vi "Begin.vi"(8 "error in":errorcluster) -> (0 "error out":errorcluster)   [LabVIEW 2016]
doc: "Called before other user functions, this VI is expected to open initial I/O refnums, load in file data, and do all program initialization. Notice that the <B>error out</B> terminal is simply used for data flow. Wiring it to other structures or subVIs ensures that this VI runs first."
uses:
  <vilib>/Rock Robotics/WPI/Joystick/WPI_JoystickDeviceEnum.ctl
  <vilib>/Rock Robotics/SystemInterfaces/DIO/FPGA_DIOPWMChannel.ctl
  <vilib>/Rock Robotics/WPI/SafetyOutput/WPI_SafetyOutputConfigMenu.ctl
  <vilib>/Rock Robotics/SystemInterfaces/DIO/FPGA_DIOChannel.ctl
  <vilib>/Rock Robotics/WPI/Solenoid/WPI_SolenoidChannel.ctl
  <vilib>/Rock Robotics/SystemInterfaces/i2clib/i2c_bus.ctl
  <vilib>/Rock Robotics/WPI/SerialPort/WPI_SerialPort.ctl
  <vilib>/Rock Robotics/SystemInterfaces/AI/FPGA_AIChannel.ctl
  <vilib>/Rock Robotics/WPI/Counter/WPI_CounterDigitalInputToDigitalSource.vi
  <vilib>/Rock Robotics/WPI/MotorControl/WPI_MotorControlOpen SPARK.vi
  <vilib>/Rock Robotics/WPI/Solenoid/WPI_SolenoidOpenDouble.vi
  <vilib>/Rock Robotics/WPI/RobotDrive/WPI_RobotDriveOpen2MotorWithSPARK.vi
  Robot Global Reference.vi
  Robot Values.vi
  Robot Global Data.vi
  <vilib>/Rock Robotics/WPI/DriverStation/WPI_DriverStationRobotMode2.ctl
  <vilib>/Rock Robotics/Network Tables/NT Write String Array.vi
  <vilib>/Rock Robotics/WPI/RobotDrive/WPI_RobotDriveOpen2MotorWithTalon.vi
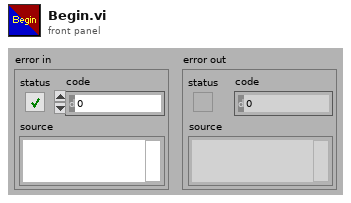
[diagram p1: front panel]
types:
  T1 = typedef "FPGA_AIChannel.ctl" = enum8{"AI 0", "AI 1", "AI 2", "AI 3", "AI MXP 0", "AI MXP 1", "AI MXP 2", "AI MXP 3", "Invalid"}
  T2 = typedef "WPI_SerialPort.ctl" = enum16{"Onboard RS-232", "MXP TTL", "USB 1", "USB 2"}
  T3 = typedef "WPI_SolenoidChannel.ctl" = enum8{"Solenoid 0", "Solenoid 1", "Solenoid 2", "Solenoid 3", "Solenoid 4", "Solenoid 5", "Solenoid 6", "Solenoid 7", "Invalid"}
  T4 = typedef "i2c_bus.ctl" = enum16{"I2C On-Board", "I2C MXP", "Invalid"}
  T5 = typedef "FPGA_DIOChannel.ctl" = enum8{"DIO 0", "DIO 1", "DIO 2", "DIO 3", "DIO 4", "DIO 5", "DIO 6", "DIO 7", "DIO 8", "DIO 9", "DIO MXP 0", "DIO MXP 1", "DIO MXP 2", "DIO MXP 3", "DIO MXP 4", "DIO MXP 5", "DIO MXP 6", "DIO MXP 7", "DIO MXP 8", "DIO MXP 9", "DIO MXP 10", "DIO MXP 11", "DIO MXP 12", "DIO MXP 13", "DIO MXP 14", "DIO MXP 15", "SPI Port CS1", "SPI Port CS2", "SPI Port CS3", "SPI Port MISO", "SPI Port MOSI", "Invalid"}
  T6 = typedef "FPGA_DIOPWMChannel.ctl" = enum8{"PWM 0", "PWM 1", "PWM 2", "PWM 3", "PWM 4", "PWM 5", "PWM 6", "PWM 7", "PWM 8", "PWM 9", "PWM MXP 0", "PWM MXP 1", "PWM MXP 2", "PWM MXP 3", "PWM MXP 4", "PWM MXP 5", "PWM MXP 6", "PWM MXP 7", "PWM MXP 8", "PWM MXP 9", "Invalid"}
  T7 = typedef "WPI_SafetyOutputConfigMenu.ctl" = enum16{"Enable", "Disable"}
  T8 = typedef "WPI_JoystickDeviceEnum.ctl" = enum16{"USB 0", "USB 1", "USB 2", "USB 3", "USB 4", "USB 5"}
  T9 = typedef "WPI_SerialPortRef.ctl" = cluster{"DevStatus":errorcluster, "Serial Port Name":refnum<visa-resource-name>}
  T10 = typedef "WPI_AnalogChannelDevRef.ctl" = cluster{"DevStatus":errorcluster, "Analog Channel":T1}
  T11 = typedef "WPI_DigitalInputDevRef.ctl" = cluster{"DevStatus":errorcluster, "DIO Channel":T5}
  T12 = typedef "FPGA_CounterEncoderSourceConvertionLVSourceType.ctl" = cluster{"DevStatus":errorcluster, "AnalogTriggerMode?":bool, "DigitalMode":cluster{"DIO Channel":T13}, "AnalogTriggerMode":cluster{"AnalogTriggerIndex":T14, "OutputType":T15}}
  T13 = typedef "FPGA_DIODigitalSourceChannel.ctl" = enum8{"DIO 0", "DIO 1", "DIO 2", "DIO 3", "DIO 4", "DIO 5", "DIO 6", "DIO 7", "DIO 8", "DIO 9", "DIO MXP 0", "DIO MXP 1", "DIO MXP 2", "DIO MXP 3", "DIO MXP 4", "DIO MXP 5", "DIO MXP 6", "DIO MXP 7", "DIO MXP 8", "DIO MXP 9", "DIO MXP 10", "DIO MXP 11", "DIO MXP 12", "DIO MXP 13", "DIO MXP 14", "DIO MXP 15", "Disabled"}
  T14 = typedef "FPGA_AnalogTriggerIndex.ctl" = enum8{"Trig 0", "Trig 1", "Trig 2", "Trig 3", "Trig 4", "Trig 5", "Trig 6", "Trig 7", "Invalid"}
  T15 = typedef "FPGA_AnalogTriggerOutType.ctl" = enum16{"InWindow", "TriggerState", "Rising", "Falling"}
  T16 = typedef "WPI_I2CDevRef.ctl" = cluster{"DevStatus":errorcluster, "Device Address":u8, "Handle":i32, "I2C Bus":T4}
  T17 = typedef "WPI_SolenoidDevRef.ctl" = cluster{"DevStatus":errorcluster, "Pneumatics Control Module":u8, "Forward Solenoid Channel":T3, "Reverse Solenoid Channel":T3}
  T18 = typedef "WPI_EncoderDevRef.ctl" = cluster{"DevStatus":errorcluster, "EncoderIndex":T19, "CounterIndex":T20, "DistancePerCount":dbl, "Decoding Type":T21}
  T19 = typedef "FPGA_EncoderIdx.ctl" = enum8{"Enc 0", "Enc 1", "Enc 2", "Enc 3", "Enc 4", "Enc 5", "Enc 6", "Enc 7", "Invalid"}
  T20 = typedef "FPGA_CounterCtrSystemIndex.ctl" = enum8{"Ctr 0", "Ctr 1", "Ctr 2", "Ctr 3", "Ctr 4", "Ctr 5", "Ctr 6", "Ctr 7", "Invalid"}
  T21 = typedef "WPI_EncoderType.ctl" = enum16{"1x", "2x", "4x"}
  T22 = typedef "WPI_MotorControlDeviceRef.ctl" = cluster{"DeviceStatus":errorcluster, "Type":T23, "PWM":cluster{"PWM Channel":T6, "DeadBand":T24}, "CAN":cluster{"Device Number":u8, "SetOutput VI Ref":variant, "GetOutput VI Ref":variant, "Enable VI Ref":variant, "Disable VI Ref":variant, "Data":variant}, "Invert":bool}
  T23 = typedef "WPI_MotorControlType.ctl" = enum16{"PWM", "CAN"}
  T24 = typedef "WPI_PWMDeadband.ctl" = cluster{"Name":string, "maxPositivePwm":i32, "minPositivePwm":i32, "centerPwm":i32, "maxNegativePwm":i32, "minNegativePwm":i32, "angularRange":u16}
  T25 = typedef "WPI_RobotDriveDevRef.ctl" = cluster{"DevStatus":errorcluster, "Motors[]":T22[], "Square Inputs":bool, "Max Output":dbl}
  T26 = typedef "WPI_JoystickDevRef.ctl" = cluster{"Device":T8}
  T27 = typedef "Robot Values.ctl" = cluster{"Robot Drive":cluster{"Left Motor Power":dbl, "Right Motor Power":dbl, "Left Encoder Value":dbl, "Right Encoder Value":dbl, "High Gear?":bool, "PTO?":bool}, "Sensors":cluster{"Gyro Angle":u16, "Recalibrate Gyro":bool, "Reset Gyro":bool, "Ultrasonic":dbl}, "Shooter":cluster{"Prep Wheels":bool, "Shoot":bool, "Left Shooter Wheel Speed":dbl, "Wheels Moving":bool, "Shooter Prepped":bool, "Shooter RPS SP":dbl, "Shooting?":bool, "Left Shooter Wheel Power":dbl, "Right Shooter Wheel Power":dbl, "Acquisition Conveyor Power":dbl, "Hopper Beater Bar Power":dbl, "Filtered Left Shooter Speed":dbl, "Acquisition Motor Power":dbl, "Joystick Add":dbl, "D-Pad Add":dbl, "Shooter Use PID?":bool}, "Robot States":cluster{"Drive mode":string, "Alliance":T28, "Position":T29}, "Gear":cluster{"Ejection Active":bool}}
  T28 = typedef "WPI_DriverStationAllianceInfo.ctl" = enum16{"Red", "Blue", "Invalid"}
  T29 = typedef "WPI_DriverStationPositionInfo.ctl" = enum16{"1", "2", "3"}
  T30 = typedef "WPI_DriverStationRobotMode2.ctl" = enum16{"Autonomous Disabled", "Autonomous Enabled", "Teleop Disabled", "Teleop Enabled", "Disconnected", "Finish", "Test Disabled", "Test Enabled", "Emergency Stopped"}
  T31 = typedef "Joystick Reference.ctl" = cluster{"Driver Joystick":T26, "Operator Joystick":T26}
  T32 = typedef "Drive Reference.ctl" = cluster{"RobotDriveDevRef":T25, "Drive PTO Solenoid":T17, "High Gear Solenoid":T17}
  T33 = typedef "Sensor Reference.ctl" = cluster{"LeftMotorEncoderRef":T18, "RightMotorEncoderRef":T18, "I2C Gyro":T16, "Left Shooter Wheel Encoder":T18, "Ultrasonic AIDeviceRef":T10}
  T34 = typedef "Shoot Reference.ctl" = cluster{"Shooter Wheel Left":T22, "Shooter Wheel Right":T22, "Acquisition Conveyor Motor DevRef":T22, "Hopper Beater Bar Motor DevRef":T22}
  T35 = typedef "Gear Reference.ctl" = cluster{"Gear Ejection Cylinder":T17, "Door Ejection Cylinder":T17}
  T36 = typedef "Light Reference.ctl" = cluster{"SerialPortRef":T9}
  T37 = cluster{"Joystick Reference":T31, "Drive Reference":T32, "Sensor Reference":T33, "Shoot + Aquisition Reference":T34, "Gear Reference":T35, "Acquisition Conveyor Motor DevRef":T22, "Lights":T36}
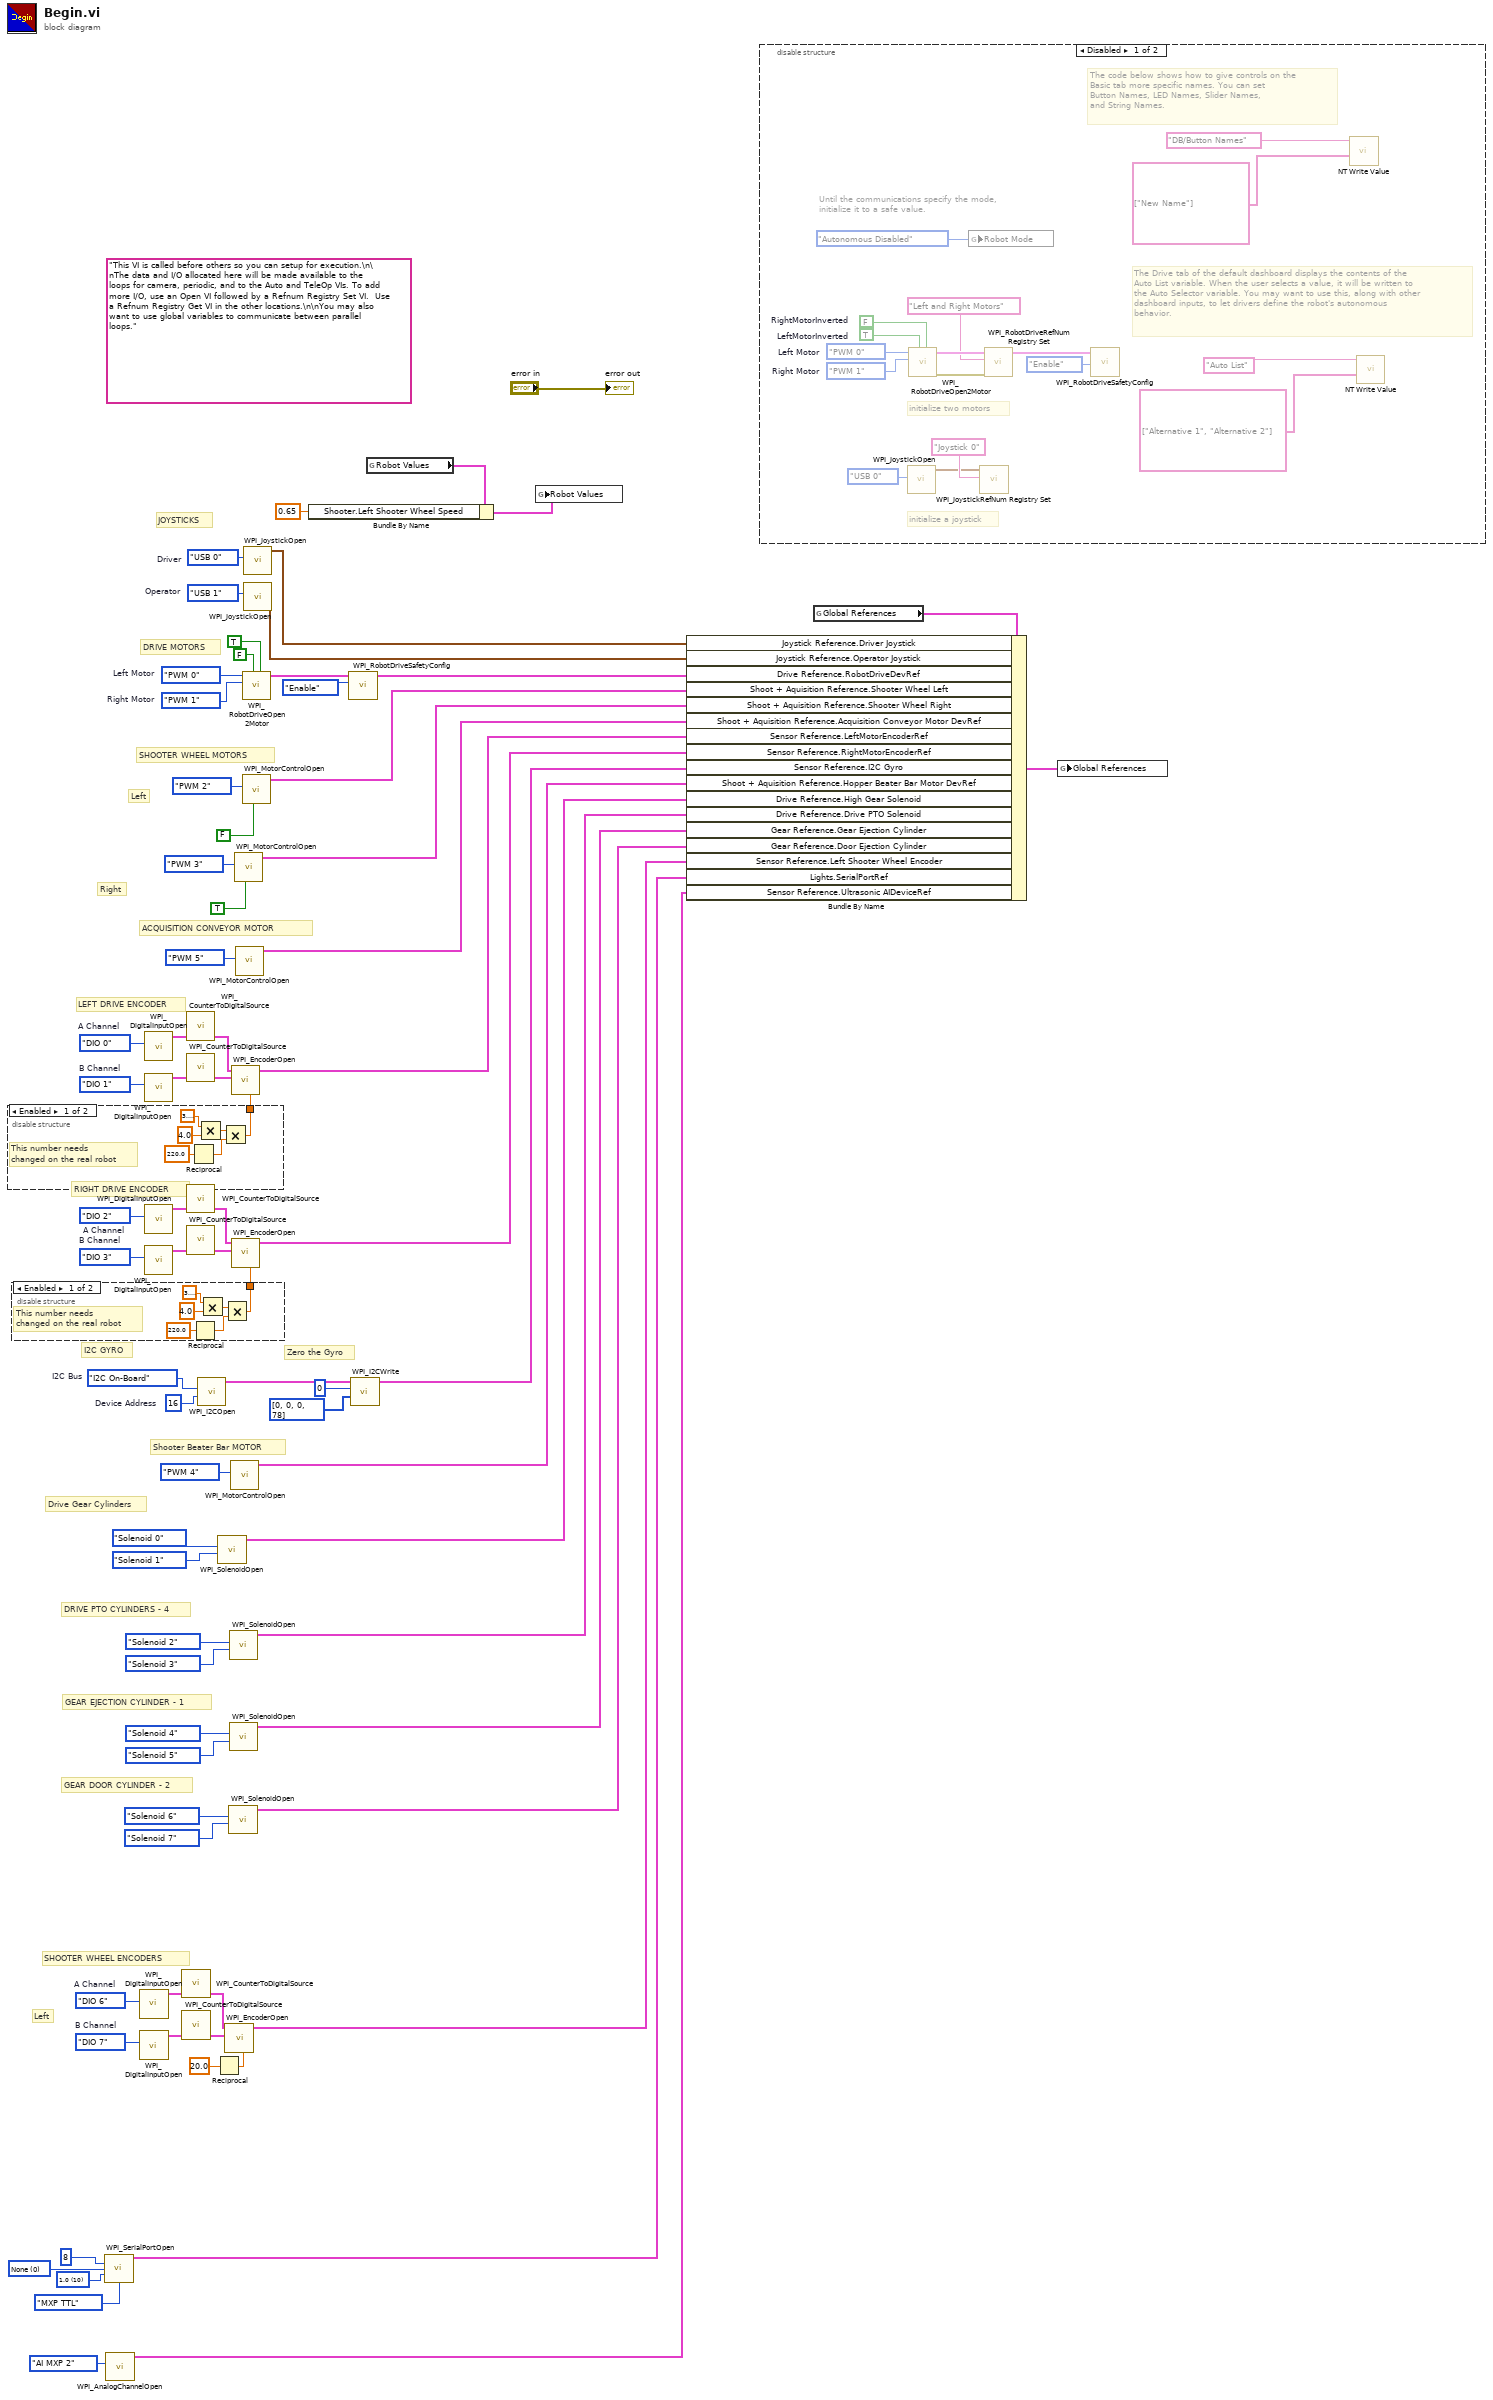
[diagram p0: block diagram]
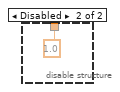
[diagram p2: hidden frame]
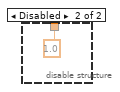
[diagram p3: hidden frame]
diagram:
  w6 = u16 0 items=["None", "Odd", "Even", "Mark", "Space"] ("Parity")
  w7 = u16 10 items=["1.0"=10, "1.5"=15, "2.0"=20] ("Stop Bits")
  w26 = u8 16  # Device Address
  w27 = i2c_bus."I2C On-Board"  # I2C Bus
  w34 = FPGA_DIOChannel."DIO 7"  # B Channel
  w33 = FPGA_DIOChannel."DIO 6"  # A Channel
  w54 = FPGA_DIOChannel."DIO 3"  # B Channel
  w55 = FPGA_DIOChannel."DIO 2"  # A Channel
  w65 = FPGA_DIOChannel."DIO 1"  # B Channel
  w64 = FPGA_DIOChannel."DIO 0"  # A Channel
  w69 = FPGA_DIOPWMChannel."PWM 1"  # Right Motor
  w70 = FPGA_DIOPWMChannel."PWM 0"  # Left Motor
  w73 = WPI_JoystickDeviceEnum."USB 1"  # Operator
  w74 = WPI_JoystickDeviceEnum."USB 0"  # Driver
  (unwired) "This VI is called before others so you can setup for execution.\n\nThe data and I/O allocated here will be made available to the loops for camera, periodic, and to the Auto and TeleOp VIs. To add more I/O, use an Open VI followed by a Refnum Registry Set VI.  Use a Refnum Registry Get VI in the other locations.\n\nYou may also want to use global variables to communicate between parallel loops."
  # "RIGHT DRIVE ENCODER"
  # "Drive Gear Cylinders"
  # "Right"
  # "Left"
  # "Left"
  # "Zero the Gyro"
  # "SHOOTER WHEEL ENCODERS"
  # "GEAR DOOR CYLINDER - 2"
  # "GEAR EJECTION CYLINDER - 1"
  # "DRIVE PTO CYLINDERS - 4"
  # "Shooter Beater Bar MOTOR"
  # "I2C GYRO"
  # "ACQUISITION CONVEYOR MOTOR"
  # "SHOOTER WHEEL MOTORS"
  # "LEFT DRIVE ENCODER"
  # "DRIVE MOTORS"
  # "JOYSTICKS"
  n1 = disable-structure shown="Enabled" {
    disable-tunnel: [w83 1.0 ("DistancePerCount")] -> w11
    frame Enabled {
      # "This number needs \nchanged on the real robot"
      n2 = Reciprocal(x=220.0) -> (1/x=w78:dbl)
      n3 = Multiply(x=3.141592653589793, y=4.0 ("x")) -> (x*y=w81:dbl)
      n4 = Multiply(x=w81, y=w78) -> (x*y=w83:dbl)
    }
    frame Disabled {
    }
  }
  n5 = disable-structure shown="Enabled" {
    disable-tunnel: [w90 1.0 ("DistancePerCount")] -> w20
    frame Enabled {
      # "This number needs \nchanged on the real robot"
      n6 = Reciprocal(x=220.0) -> (1/x=w89:dbl)
      n7 = Multiply(x=3.141592653589793, y=4.0 ("x")) -> (x*y=w87:dbl)
      n8 = Multiply(x=w87, y=w89) -> (x*y=w90:dbl)
    }
    frame Disabled {
    }
  }
  n9 = call <vilib>:"WPI_SerialPortOpen.vi"("Data Bits"=u16 8, "Parity"=w6, "Stop Bits"=w7, "Serial Port"=WPI_SerialPort."MXP TTL") -> ("SerialPortRef"=w3:T9)  [unwired: 10 in, 1 out]
  n10 = call <vilib>:"WPI_AnalogChannelOpen.vi"("Analog Channel"=FPGA_AIChannel."AI MXP 2") -> ("AIDeviceRef"=w1:T10)  [unwired: 9 in, 1 out]
  n11 = call <vilib>:"WPI_DigitalInputOpen.vi"("DIO Channel"=w33) -> ("DigitalInputDevRef"=w30:T11)  [unwired: 1 in, 9 out]
  n12 = call <vilib>:"WPI_DigitalInputOpen.vi"("DIO Channel"=w34) -> ("DigitalInputDevRef"=w31:T11)  [unwired: 1 in, 9 out]
  n13 = call <vilib>:"WPI_DigitalInputOpen.vi"("DIO Channel"=w64) -> ("DigitalInputDevRef"=w61:T11)  [unwired: 1 in, 9 out]
  n14 = call <vilib>:"WPI_DigitalInputOpen.vi"("DIO Channel"=w65) -> ("DigitalInputDevRef"=w62:T11)  [unwired: 1 in, 9 out]
  n15 = call <vilib>:"WPI_DigitalInputOpen.vi"("DIO Channel"=w55) -> ("DigitalInputDevRef"=w58:T11)  [unwired: 1 in, 9 out]
  n16 = call <vilib>:"WPI_DigitalInputOpen.vi"("DIO Channel"=w54) -> ("DigitalInputDevRef"=w57:T11)  [unwired: 1 in, 9 out]
  n17 = call-poly <vilib>:"WPI_CounterToDigitalSource.vi"("DigitalInputDevRef"=w30) -> ("Digital Source"=w29:T12)  [unwired: 6 out]
  n18 = call-poly <vilib>:"WPI_CounterToDigitalSource.vi"("DigitalInputDevRef"=w31) -> ("Digital Source"=w32:T12)  [unwired: 6 out]
  n19 = call-poly <vilib>:"WPI_CounterToDigitalSource.vi"("DigitalInputDevRef"=w61) -> ("Digital Source"=w60:T12)  [unwired: 6 out]
  n20 = call-poly <vilib>:"WPI_CounterToDigitalSource.vi"("DigitalInputDevRef"=w62) -> ("Digital Source"=w63:T12)  [unwired: 6 out]
  n21 = call-poly <vilib>:"WPI_CounterToDigitalSource.vi"("DigitalInputDevRef"=w58) -> ("Digital Source"=w59:T12)  [unwired: 6 out]
  n22 = call-poly <vilib>:"WPI_CounterToDigitalSource.vi"("DigitalInputDevRef"=w57) -> ("Digital Source"=w56:T12)  [unwired: 6 out]
  n23 = call <vilib>:"WPI_I2COpen.vi"("Device Address"=w26, "I2C Bus"=w27) -> ("I2CDevRef"=w25:T16)  [unwired: 8 in, 1 out]
  n24 = Reciprocal(x=20.0) -> (1/x=w19:dbl)
  n25 = call-poly <vilib>:"WPI_SolenoidOpen.vi"("Reverse Solenoid Channel"=WPI_SolenoidChannel."Solenoid 1", "Forward Solenoid Channel"=WPI_SolenoidChannel."Solenoid 0" ("Solenoid Channel")) -> ("SolenoidDevRef"=w14:T17)  [unwired: 8 in, 1 out]
  n26 = call <vilib>:"WPI_EncoderOpen.vi"("DistancePerCount"=w19, "BSource"=w32, "ASource"=w29) -> ("EncoderDevRef"=w28:T18)  [unwired: 5 in, 3 out]
  n27 = call-poly <vilib>:"WPI_SolenoidOpen.vi"("Reverse Solenoid Channel"=WPI_SolenoidChannel."Solenoid 7", "Forward Solenoid Channel"=WPI_SolenoidChannel."Solenoid 6" ("Solenoid Channel")) -> ("SolenoidDevRef"=w35:T17)  [unwired: 8 in, 1 out]
  n28 = call-poly <vilib>:"WPI_SolenoidOpen.vi"("Reverse Solenoid Channel"=WPI_SolenoidChannel."Solenoid 3", "Forward Solenoid Channel"=WPI_SolenoidChannel."Solenoid 2" ("Solenoid Channel")) -> ("SolenoidDevRef"=w41:T17)  [unwired: 8 in, 1 out]
  n29 = call-poly <vilib>:"WPI_SolenoidOpen.vi"("Reverse Solenoid Channel"=WPI_SolenoidChannel."Solenoid 5", "Forward Solenoid Channel"=WPI_SolenoidChannel."Solenoid 4" ("Solenoid Channel")) -> ("SolenoidDevRef"=w36:T17)  [unwired: 8 in, 1 out]
  n30 = call-poly <vilib>:"WPI_MotorControlOpen.vi"("PWM Channel"=FPGA_DIOPWMChannel."PWM 4") -> ("MotorControlDeviceRef"=w45:T22)  [unwired: 9 in, 1 out]
  n31 = call <vilib>:"WPI_EncoderOpen.vi"("DistancePerCount"=w11, "BSource"=w63, "ASource"=w60) -> ("EncoderDevRef"=w47:T18)  [unwired: 5 in, 3 out]
  n32 = call <vilib>:"WPI_EncoderOpen.vi"("DistancePerCount"=w20, "BSource"=w56, "ASource"=w59) -> ("EncoderDevRef"=w46:T18)  [unwired: 5 in, 3 out]
  n33 = call-poly <vilib>:"WPI_MotorControlOpen.vi"("Invert"=TRUE, "PWM Channel"=FPGA_DIOPWMChannel."PWM 3") -> ("MotorControlDeviceRef"=w50:T22)  [unwired: 8 in, 1 out]
  n34 = call-poly <vilib>:"WPI_MotorControlOpen.vi"("PWM Channel"=FPGA_DIOPWMChannel."PWM 5") -> ("MotorControlDeviceRef"=w48:T22)  [unwired: 9 in, 1 out]
  n35 = call-poly <vilib>:"WPI_RobotDriveOpen2Motor.vi"("Right Motor Inverted"=TRUE, "Left Motor Inverted"=FALSE, "Right Motor"=w69, "Left Motor"=w70) -> ("RobotDriveDevRef"=w68:T25)  [unwired: 6 in, 1 out]
  n36 = call-poly <vilib>:"WPI_MotorControlOpen.vi"("Invert"=FALSE, "PWM Channel"=FPGA_DIOPWMChannel."PWM 2") -> ("MotorControlDeviceRef"=w52:T22)  [unwired: 8 in, 1 out]
  n37 = call <vilib>:"WPI_JoystickOpen.vi"("JoystickDevice"=w74) -> ("JoystickDevRef"=w72:T26)  [unwired: 10 in]
  n38 = call <vilib>:"WPI_JoystickOpen.vi"("JoystickDevice"=w73) -> ("JoystickDevRef"=w71:T26)  [unwired: 10 in]
  n39 = call <vilib>:"WPI_RobotDriveSafetyConfig.vi"("mode"=WPI_SafetyOutputConfigMenu."Enable", "RobotDriveDevRef"=w68) -> ("RobotDriveDevRef"=w66:T25)  [unwired: 8 in, 1 out]
  n40 = call <vilib>:"WPI_I2CWrite.vi"("I2CDataToSend"=u8[] [0, 0, 0, 78], "I2CRegister"=u8 0, "I2CDevRef"=w25) -> ("I2CDevRef"=w24:T16)  [unwired: 7 in, 1 out]
  n41 = global read "Robot Values.vi" "Robot Values"() -> (w9:T27)
  n42 = Bundle By Name(cluster=w9, "Shooter.Left Shooter Wheel Speed"=0.65) -> (w10:T27)
  n43 = global write "Robot Values.vi" "Robot Values"(w10) -> ()
  n44 = disable-structure shown="Disabled" {
    frame Disabled {
      w102 = FPGA_DIOPWMChannel."PWM 1"  # Right Motor
      w103 = FPGA_DIOPWMChannel."PWM 0"  # Left Motor
      w107 = TRUE  # LeftMotorInverted
      w108 = FALSE  # RightMotorInverted
      # "The Drive tab of the default dashboard displays the contents of the\nAuto List variable. When the user selects a value, it will be written to\nthe Auto Selector variable. You may want to use this, along with other\ndashboard inputs, to let drivers define the robot's autonomous\nbehavior."
      # "The code below shows how to give controls on the\nBasic tab more specific names. You can set\nButton Names, LED Names, Slider Names,\nand String Names."
      # "initialize a joystick"
      # "Until the communications specify the mode,\ninitialize it to a safe value."
      # "initialize two motors"
      n45 = call <vilib>:"WPI_JoystickOpen.vi"("JoystickDevice"=WPI_JoystickDeviceEnum."USB 0") -> ("JoystickDevRef"=w97:T26)  [unwired: 10 in]
      n46 = call-poly <vilib>:"WPI_RobotDriveOpen2Motor.vi"("Right Motor Inverted"=w108, "Left Motor Inverted"=w107, "Right Motor"=w102, "Left Motor"=w103) -> ("error out"=w104:errorcluster, "RobotDriveDevRef"=w106:T25)  [unwired: 1 in, 5 out]
      n47 = global write "Robot Global Data.vi" "Robot Mode"(WPI_DriverStationRobotMode2."Autonomous Disabled" ("Robot Mode")) -> ()
      n48 = call <vilib>:"WPI_JoystickRefNum Registry Set.vi"("refnum name"="Joystick 0", "JoystickDevRef"=w97) -> ()  [unwired: 8 in, 2 out]
      n49 = call <vilib>:"WPI_RobotDriveRefNum Registry Set.vi"("error in (no error)"=w104, "refnum name"="Left and Right Motors", "RobotDriveDevRef"=w106) -> ("RobotDriveDevRef"=w101:T25)  [unwired: 1 in, 7 out]
      n50 = call <vilib>:"WPI_RobotDriveSafetyConfig.vi"("mode"=WPI_SafetyOutputConfigMenu."Enable", "RobotDriveDevRef"=w101) -> ()  [unwired: 8 in, 2 out]
      n51 = call-poly <vilib>:"NT Write Value.vi"("String Array"=string[] ["New Name"], "Name"="DB/Button Names") -> ()  [unwired: 9 in, 1 out]
      n52 = call-poly <vilib>:"NT Write Value.vi"("String Array"=string[] ["Alternative 1", "Alternative 2"], "Name"="Auto List") -> ()  [unwired: 9 in, 1 out]
    }
    frame Enabled {
    }
  }
  n53 = global read "Robot Global Reference.vi" "Global References"() -> (w76:T37)
  n54 = Bundle By Name(cluster=w76, "Joystick Reference.Driver Joystick"=w72, "Joystick Reference.Operator Joystick"=w71, "Drive Reference.RobotDriveDevRef"=w66, "Shoot + Aquisition Reference.Shooter Wheel Left"=w52, "Shoot + Aquisition Reference.Shooter Wheel Right"=w50, "Shoot + Aquisition Reference.Acquisition Conveyor Motor DevRef"=w48, "Sensor Reference.LeftMotorEncoderRef"=w47, "Sensor Reference.RightMotorEncoderRef"=w46, "Sensor Reference.I2C Gyro"=w24, "Shoot + Aquisition Reference.Hopper Beater Bar Motor DevRef"=w45, "Drive Reference.High Gear Solenoid"=w14, "Drive Reference.Drive PTO Solenoid"=w41, "Gear Reference.Gear Ejection Cylinder"=w36, "Gear Reference.Door Ejection Cylinder"=w35, "Sensor Reference.Left Shooter Wheel Encoder"=w28, "Lights.SerialPortRef"=w3, "Sensor Reference.Ultrasonic AIDeviceRef"=w1) -> (w75:T37)
  n55 = global write "Robot Global Reference.vi" "Global References"(w75) -> ()
  "error out" <- "error in"
